vi "RT Main.vi"() -> ()   [LabVIEW 2021]
doc: "This example publishes data acquired from the myRIO device using shared variables. These shared variables can be accessed with an iPad running the sample dashboard."
uses:
  <vilib>/myRIO/Instrument Drivers/Utilities/Utilities.lvlib
  <vilib>/myRIO/Instrument Drivers/Onboard IO/AI/AI.lvlib
  <vilib>/myRIO/Instrument Drivers/Onboard IO/AO/AO.lvlib
  <vilib>/myRIO/Instrument Drivers/Onboard IO/DIO/DIO.lvlib
  <vilib>/ptbypt/NI_PtbyPt.lvlib
  <vilib>/Platform/TimedLoop/XDataNode/XDataNode.xnode
  <vilib>/Platform/TimedLoop/XDataNode/nitl_modes.ctl
  <vilib>/Platform/TimedLoop/XDataNode/XDNodeRunTimeDep.lvlib
  <vilib>/Platform/TimedLoop/XDataNode/wakeup.ctl
  <vilib>/Platform/TimedLoop/XDataNode/timing_clust.ctl
  <vilib>/myRIO/Instrument Drivers/Onboard IO/AI/vis/myRIO AI Open.xnode
  <vilib>/myRIO/Common/Instrument Driver Framework/Utilities/typedefs/Hardware Version Enum.ctl
  <vilib>/myRIO/Common/Instrument Driver Framework/Utilities/typedefs/Generic FPGA Reference.ctl
  <vilib>/myRIO/Common/Instrument Driver Framework/Utilities/typedefs/myRIO v1.0 Reference.ctl
  <vilib>/myRIO/Common/Instrument Driver Framework/Utilities/typedefs/myRIO Generic Hardware Reference.ctl
  <vilib>/myRIO/Common/Instrument Driver Framework/myRIO v1.0/AI/typedefs/AI Channels Enum.ctl
  <vilib>/myRIO/Common/Instrument Driver Framework/myRIO v1.0/AI/typedefs/AI Channels List.ctl
  <vilib>/myRIO/Common/Instrument Driver Framework/Utilities/typedefs/Analog Scaling Constants.ctl
  <vilib>/myRIO/Common/Instrument Driver Framework/Utilities/typedefs/Analog Scaling Constants List.ctl
  <vilib>/myRIO/Instrument Drivers/Onboard IO/AI/typedefs/AI Reference.ctl
  <vilib>/userdefined/High Color/nirio_resource_hc.ctl
  <vilib>/myRIO/Instrument Drivers/Onboard IO/AO/vis/myRIO AO Open.xnode
  <vilib>/myRIO/Common/Instrument Driver Framework/myRIO v1.0/AO/typedefs/AO Channels Enum.ctl
  <vilib>/myRIO/Common/Instrument Driver Framework/myRIO v1.0/AO/typedefs/AO Channels List.ctl
  <vilib>/myRIO/Instrument Drivers/Onboard IO/AO/typedefs/AO Reference.ctl
  <vilib>/myRIO/Instrument Drivers/Onboard IO/DIO/vis/myRIO DIO Open.xnode
  <vilib>/myRIO/Common/Instrument Driver Framework/myRIO v1.0/DIO/typedefs/DIO Channels Enum.ctl
  <vilib>/myRIO/Common/Instrument Driver Framework/myRIO v1.0/DIO/typedefs/DIO Channels List.ctl
  <vilib>/myRIO/Instrument Drivers/Onboard IO/DIO/typedefs/DIO Reference.ctl
  <vilib>/myRIO/Common/Instrument Driver Framework/myRIO v1.0/DIO/vis/myRIO v1.1 Open DIO.vi
  <vilib>/myRIO/Express VI/Onboard IO/AI/AI Express VI.xnode
  <vilib>/myRIO/Express VI/Onboard IO/AO/AO Express VI.xnode
  <vilib>/myRIO/Express VI/Onboard Devices/LED/LED Express VI.xnode
  <vilib>/myRIO/Common/Instrument Driver Framework/myRIO v1.0/AI/vis/myRIO v1.1 Open AI.vi
  <vilib>/myRIO/Common/Instrument Driver Framework/myRIO v1.0/AO/vis/myRIO v1.1 Open AO.vi
  <vilib>/myRIO/Common/Instrument Driver Framework/Utilities/vis/Is FPGA Ref Available.vi
  <vilib>/myRIO/Express VI/Onboard Devices/Accelerometer/Accelerometer Express VI.xnode
  <vilib>/myRIO/Instrument Drivers/Onboard Devices/Accelerometer/Accelerometer.lvlib
  <vilib>/myRIO/Common/Instrument Driver Framework/myRIO v1.0/Accelerometer/typedefs/Accelerometer Channels Enum.ctl
  <vilib>/myRIO/Common/Instrument Driver Framework/myRIO v1.0/Accelerometer/typedefs/Accelerometer Channels List.ctl
  <vilib>/myRIO/Instrument Drivers/Onboard Devices/Accelerometer/typedefs/Accelerometer Reference.ctl
  <vilib>/myRIO/Instrument Drivers/Onboard Devices/Accelerometer/vis/myRIO Accelerometer Open.xnode
  <vilib>/myRIO/Common/Instrument Driver Framework/myRIO v1.0/Accelerometer/vis/myRIO v1.1 Open Accelerometer.vi
panel:
  out "error out":errorcluster
  in  "stop":bool
  in  "Tab Control":T1(tab)
  out "LED3":bool
  out "LED2":bool
  out "LED1":bool
  out "LED0":bool
  out "Audio":waveform(dbl)[](graph)
  out "Accelerometer":waveform(dbl)[](graph)
  out "DIO.A":waveform(u8)(graph)
  out "AIO.A":waveform(dbl)[](graph)
  out "DIO.A Input/Output":enum16{"Input", "Output"}(ring)
  out "DIO Channel.A":u16(ring) items=["A/DIO0", "A/DIO1", "A/DIO2", "A/DIO3", "A/DIO4", "A/DIO5", "A/DIO6", "A/DIO7", "A/DIO8", "A/DIO9", "A/DIO10", "A/DIO11", "A/DIO12", "A/DIO13", "A/DIO14", "A/DIO15"]
  out "AO Channel.A":u16(ring) items=["A/AO0", "A/AO1"]
  out "AI Channel.A":u16(ring) items=["A/AI0", "A/AI1", "A/AI2", "A/AI3"]
  out "AIO.B":waveform(dbl)[](graph)
  out "DIO.B Input/Output":enum16{"Input", "Output"}(ring)
  out "DIO Channel.B":u16(ring) items=["B/DIO0", "B/DIO1", "B/DIO2", "B/DIO3", "B/DIO4", "B/DIO5", "B/DIO6", "B/DIO7", "B/DIO8", "B/DIO9", "B/DIO10", "B/DIO11", "B/DIO12", "B/DIO13", "B/DIO14", "B/DIO15"]
  out "AO Channel.B":u16(ring) items=["B/AO0", "B/AO1"]
  out "AI Channel.B":u16(ring) items=["B/AI0", "B/AI1", "B/AI2", "B/AI3"]
  out "DIO.B":waveform(u8)(graph)
  out "AIO.C":waveform(dbl)[](graph)
  out "DIO.C":waveform(u8)(graph)
  out "DIO.C Input/Output":enum16{"Input", "Output"}(ring)
  out "DIO Channel.C":u16(ring) items=["C/DIO0", "C/DIO1", "C/DIO2", "C/DIO3", "C/DIO4", "C/DIO5", "C/DIO6", "C/DIO7"]
  out "AO Channel.C":u16(ring) items=["C/AO0", "C/AO1"]
  out "AI Channel.C":u16(ring) items=["C/AI0", "C/AI1"]
  # "Overview: This example publishes data acquired from the myRIO device using shared variables.  These shared variables can be accessed with an iPad running the sample dashboard.\nRequirements: \n1. myRIO-1900\n2. Network Variable Engine on the myRIO\n3. Data Dashboard on iPad\nInstructions:\n1. Configure Data Dashboard for your iPad as described in the readme file for this project.  (Navigate to the Project Documentation folder in the project tree and open Data Dashboard for myRIO Readme.html.)\n2. Check the myRIO target IP Address in the project and make sure the target IP Address is correct.\n3. Run this VI."
  # "There are two ways to view the shared \nvariable data published by RT Main.vi that you\nrun on the myRIO:\n--View the data on iPad: You can find detailed \ninstructions in the readme file of the Data\nDashboard for myRIO example and the help file\nof Data Dashboard.\n--View the data on PC: Run RT Main.vi on the  \nmyRIO, and run Desktop Main.vi. View the \nshared variable data in Desktop Main.vi."
  # "LED Status :"
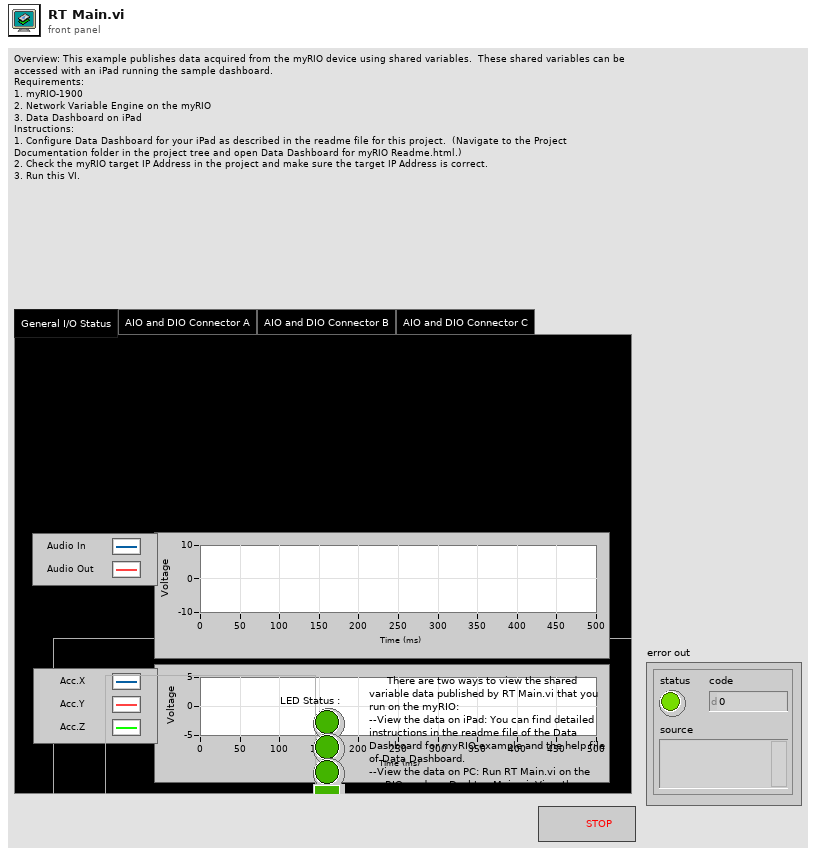
[diagram p1: front panel]
types:
  T1 = enum32{"General I/O Status", "AIO and DIO Connector A", "AIO and DIO Connector B", "AIO and DIO Connector C"}
  T2 = cluster{"read mode":enum16{"polling", "blocking"}, "write mode":enum16{"polling", "blocking"}}
  T3 = cluster{"AI.A":dbl, "AI.B":dbl, "AI.C":dbl, "AO.A":dbl, "AO.B":dbl, "AO.C":dbl, "DIO.A":u8, "DIO.B":u8, "DIO.C":u8, "Audio In":dbl, "Audio Out":dbl, "Accelerometer X":dbl, "Accelerometer Y":dbl, "Accelerometer Z":dbl, "LED0":bool, "LED1":bool, "LED2":bool, "LED3":bool}
  T4 = typedef "nirio_resource_hc.ctl" = tag
  T5 = typedef "Hardware Version Enum.ctl" = enum16{"Unknown", "myRIO-1900", "myRIO-1950", "roboRIO", "NI ELVIS RIO CM", "ELVIS III"}
  T6 = typedef "AO.lvlib/AO Reference.ctl" = cluster{"myRIO Reference":T7, "AO Channel List":T10, "AO Scaling Constant List":T12}
  T7 = typedef "myRIO Generic Hardware Reference.ctl" = cluster{"myRIO Model":T5, "myRIO Hardware Reference":T8}
  T8 = typedef "myRIO v1.0 Reference.ctl" = cluster{"Generic FPGA Reference":T9, "Allow multiple opens":bool}
  T9 = typedef "Generic FPGA Reference.ctl" = refnum<k20>
  T10 = typedef "AO Channels List.ctl" = T11[]
  T11 = typedef "AO Channels Enum.ctl" = enum16{"Not Connected", "AudioOut/Left", "AudioOut/Right", "C/AO0", "C/AO1", "A/AO0", "A/AO1", "B/AO0", "B/AO1"}
  T12 = typedef "Analog Scaling Constants List.ctl" = T13[]
  T13 = typedef "Analog Scaling Constants.ctl" = cluster{"LSB Weight (Volts)":dbl, "Offset (Volts)":dbl, "Signed?":bool}
  T14 = typedef "AI.lvlib/AI Reference.ctl" = cluster{"myRIO Reference":T7, "AI Channels List":T15, "AI Scaling Constants List":T12}
  T15 = typedef "AI Channels List.ctl" = T16[]
  T16 = typedef "AI Channels Enum.ctl" = enum16{"Not Connected", "AudioIn/Left", "AudioIn/Right", "C/AI0", "C/AI1", "A/AI0", "A/AI1", "A/AI2", "A/AI3", "A/AI4", "A/AI5", "A/AI6", "A/AI7", "B/AI0", "B/AI1", "B/AI2", "B/AI3", "B/AI4", "B/AI5", "B/AI6", "B/AI7", "AI/AI0", "AI/AI1", "AI/AI2", "AI/AI3", "A/AI0 (DIFF)", "A/AI1 (DIFF)", "A/AI2 (DIFF)", "A/AI3 (DIFF)", "B/AI0 (DIFF)", "B/AI1 (DIFF)", "B/AI2 (DIFF)", "B/AI3 (DIFF)"}
  T17 = typedef "Accelerometer.lvlib/Accelerometer Reference.ctl" = cluster{"myRIO Reference":T7, "Accelerometer Channels List":T18, "LSB Weight":dbl}
  T18 = typedef "Accelerometer Channels List.ctl" = T19[]
  T19 = typedef "Accelerometer Channels Enum.ctl" = enum16{"Not Connected", "X-Axis", "Y-Axis", "Z-Axis"}
  T20 = typedef "DIO.lvlib/DIO Reference.ctl" = cluster{"myRIO Reference":T7, "DIO Channels List":T21}
  T21 = typedef "DIO Channels List.ctl" = T22[]
  T22 = typedef "DIO Channels Enum.ctl" = enum16{"Not Connected", "C/DIO0", "C/DIO1", "C/DIO2", "C/DIO3", "C/DIO4", "C/DIO5", "C/DIO6", "C/DIO7", "A/DIO0", "A/DIO1", "A/DIO2", "A/DIO3", "A/DIO4", "A/DIO5", "A/DIO6", "A/DIO7", "A/DIO8", "A/DIO9", "A/DIO10", "A/DIO11", "A/DIO12", "A/DIO13", "A/DIO14", "A/DIO15", "A/DIO16", "A/DIO17", "A/DIO18", "A/DIO19", "B/DIO0", "B/DIO1", "B/DIO2", "B/DIO3", "B/DIO4", "B/DIO5", "B/DIO6", "B/DIO7", "B/DIO8", "B/DIO9", "B/DIO10", "B/DIO11", "B/DIO12", "B/DIO13", "B/DIO14", "B/DIO15", "B/DIO16", "B/DIO17", "B/DIO18", "B/DIO19", "LED0", "LED1", "LED2", "LED3", "Button0", "DIO/DIO0", "DIO/DIO1", "DIO/DIO2", "DIO/DIO3", "DIO/DIO4", "DIO/DIO5", "DIO/DIO6", "DIO/DIO7", "DIO/DIO8", "DIO/DIO9", "SPI/CS0", "SPI/CS1", "SPI/CS2", "SPI/CS3", "LED RADIO (Green)", "LED RADIO (Red)", "LED COMM (Green)", "LED COMM (Red)", "LED MODE (Green)", "LED MODE (Red)"}
  T23 = typedef "XDNodeRunTimeDep.lvlib/timing_clust.ctl" = cluster{"Expected End [f-1]":u64, "Actual End [f-1]":u64, "Finished Late? [f-1]":bool, "Expected End [i-1]":u64, "Actual End [i-1]":u64, "Finished Late? [i-1]":bool, "Expected Start [i]":u64, "Actual Start [i]":u64, "Expected Start [f]":u64, "Actual Start [f]":u64, "Source Name":string, "Structure Name":string, "Period":i64, "Deadline":i64, "Offset":i64, "Start":i64, "Priority":i32, "Timeout":i32, "Mode":T24, "Wakeup Reason":T25, "Error":errorcluster, "Source Type":string, "Secondary Source Type":string, "Global End Time":u64, "Global Start Time":u64, "Frame Duration":u64, "Iteration Duration":u64, "Assigned CPU":i32, "I/O Scan Engine Mode":u32}
  T24 = typedef "XDNodeRunTimeDep.lvlib/nitl_modes.ctl" = enum32{"No Change", "Process missed periods, maintain original phase", "Discard missed periods, maintain original phase", "Process missed periods, ignore original phase", "Discard missed periods, ignore original phase"}
  T25 = typedef "XDNodeRunTimeDep.lvlib/wakeup.ctl" = enum32{"Normal", "Aborted", "Asynchronous wakeup", "Timing source error", "Timed loop error", "Timeout"}
  T26 = cluster{"AI.A":dbl, "AI.B":dbl, "AI.C":dbl, "AO.A":dbl, "AO.B":dbl, "AO.C":dbl, "DIO.A":u8, "DIO.B":u8, "DIO.C":u8, "Audio In":dbl, "Audio Out":dbl, "Accelerometer X":dbl, "Accelerometer Y":dbl, "Accelerometer Z":dbl, "LED0":bool, "LED1":bool, "LED2":bool, "LED3":bool}[]
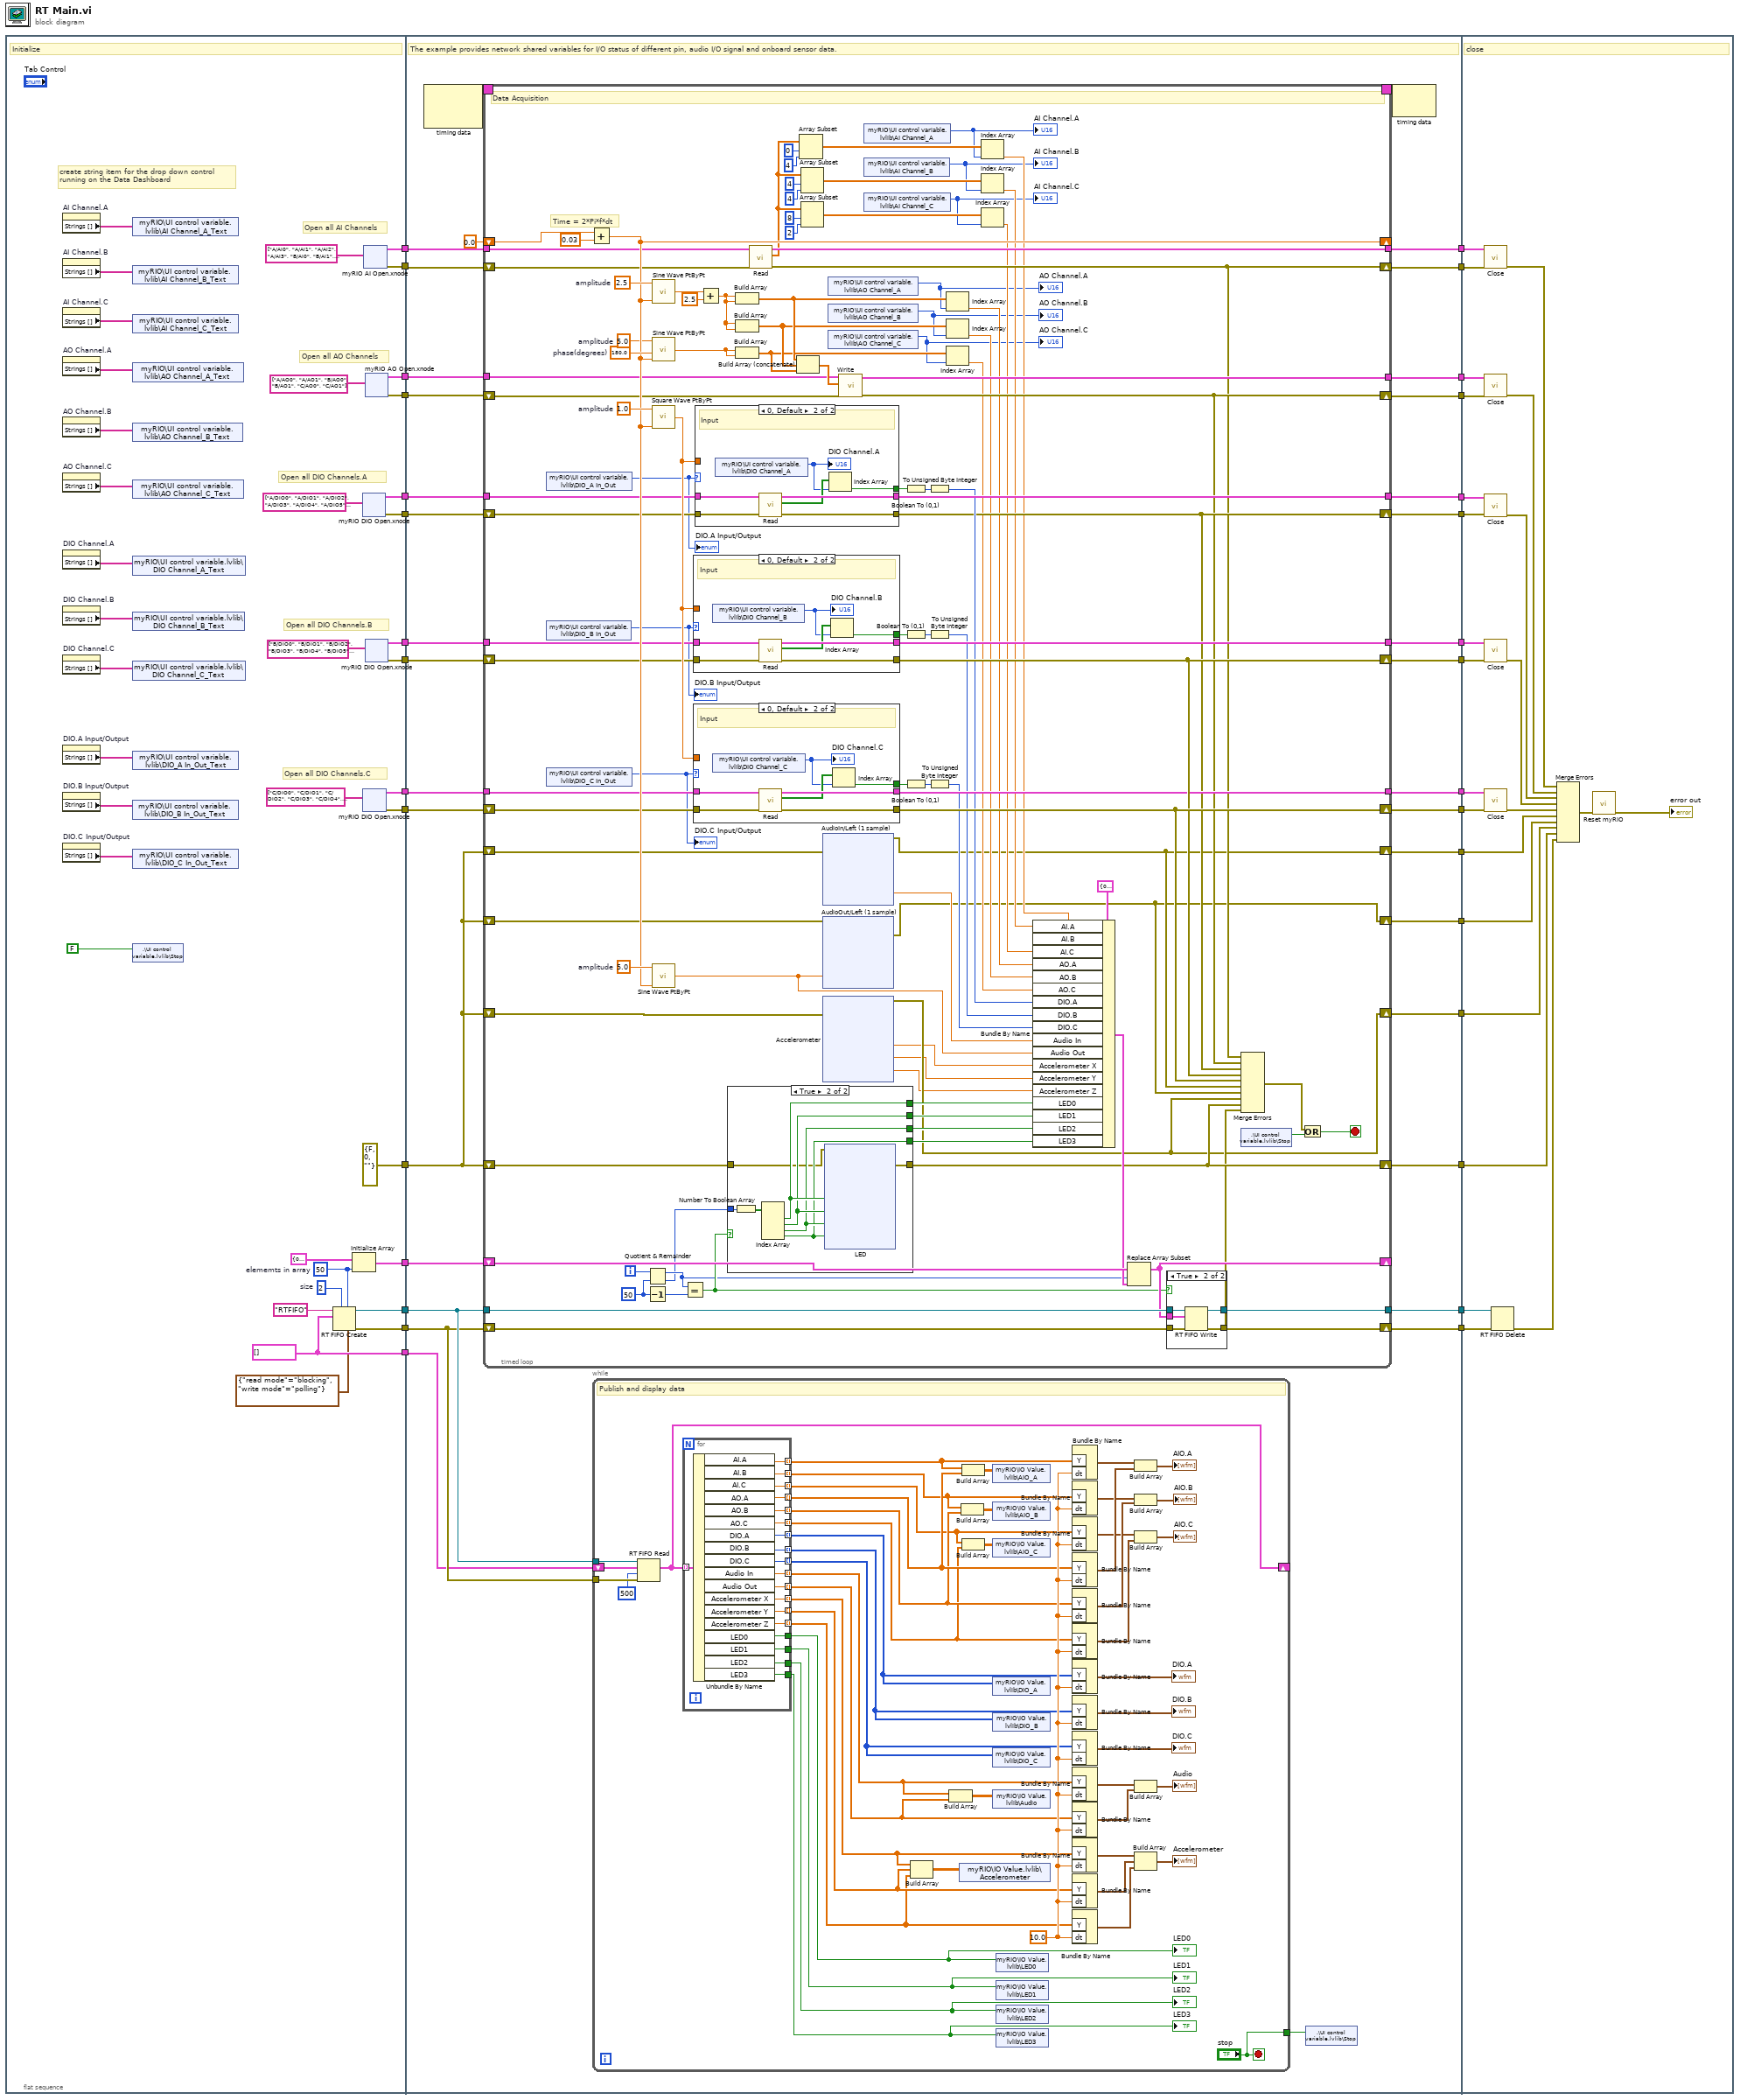
[diagram p0: block diagram]
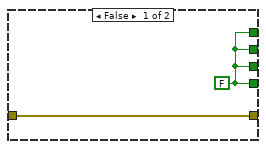
[diagram p2: hidden frame]
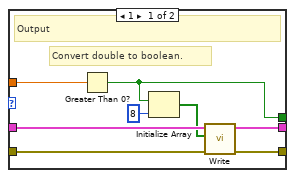
[diagram p4: hidden frame]
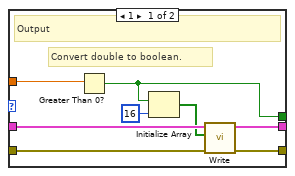
[diagram p5: hidden frame]
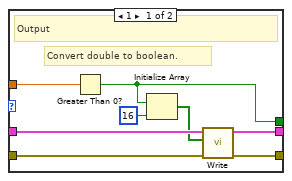
[diagram p6: hidden frame]
diagram:
  n1 = flat-sequence {
    tunnel: [errorcluster {"status"=FALSE, "code"=0, "source"=""} ("error IO")] -> w31
    tunnel: [w52] -> w14
    tunnel: [w51] -> w13
    tunnel: [w50] -> w12
    tunnel: [w49] -> w11
    tunnel: [w48] -> w10
    tunnel: [w47] -> w9
    tunnel: [w46] -> w8
    tunnel: [w45] -> w7
    tunnel: [w44] -> w6
    tunnel: [w43] -> w5
    tunnel: [w37] -> w4
    tunnel: [w36] -> w3
    tunnel: [w35] -> w2
    tunnel: [w34] -> w1
    tunnel: w31 -> [w161]
    tunnel: [w188] -> w30
    tunnel: [w155] -> w29
    tunnel: [w187] -> w28
    tunnel: [w184] -> w27
    tunnel: [w183] -> w26
    tunnel: [w182] -> w25
    tunnel: [w181] -> w24
    tunnel: [w180] -> w23
    tunnel: [w179] -> w22
    tunnel: [w178] -> w21
    tunnel: [w177] -> w20
    tunnel: [w176] -> w19
    tunnel: [w154] -> w18
    tunnel: [w175] -> w17
    tunnel: [w174] -> w16
    tunnel: [w172] -> w15
    tunnel: w14 -> [w166]
    tunnel: w13 -> [w171]
    tunnel: w12 -> [w170]
    tunnel: w11 -> [w169]
    tunnel: w10 -> [w168]
    tunnel: w9 -> [w167]
    tunnel: w8 -> [w165]
    tunnel: w7 -> [w164]
    tunnel: w6 -> [w163]
    tunnel: w5 -> [w162]
    tunnel: w4 -> [w157]
    tunnel: w3 -> [w160]
    tunnel: w2 -> [w159]
    tunnel: w1 -> [w158]
    tunnel: w30 -> [w596]
    tunnel: w29 -> [w602]
    tunnel: w28 -> [w601]
    tunnel: w27 -> [w595]
    tunnel: w26 -> [w592]
    tunnel: w25 -> [w593]
    tunnel: w24 -> [w590]
    tunnel: w23 -> [w589]
    tunnel: w22 -> [w586]
    tunnel: w21 -> [w587]
    tunnel: w20 -> [w584]
    tunnel: w19 -> [w583]
    tunnel: w18 -> [w600]
    tunnel: w17 -> [w599]
    tunnel: w16 -> [w598]
    tunnel: w15 -> [w581]
    frame #0 {
      w40 = u32 2  # size
      w39 = 50  # elememts in array
      w34 = T26 []
      # "Open all DIO Channels.C"
      # "Open all DIO Channels.B"
      # "Open all DIO Channels.A"
      # "Open all AO Channels"
      # "Open all AI Channels"
      # "create string item for the drop down control \nrunning on the Data Dashboard"
      # "Initialize"
      n2 = property on="AI Channel.A" class="Ring (strict)"() -> ("Strings []"=w69:string[])  [unwired: 2 in, 2 out]
      n3 = property on="AI Channel.B" class="Ring (strict)"() -> ("Strings []"=w68:string[])  [unwired: 2 in, 2 out]
      n4 = property on="AI Channel.C" class="Ring (strict)"() -> ("Strings []"=w67:string[])  [unwired: 2 in, 2 out]
      n5 = property on="AO Channel.A" class="Ring (strict)"() -> ("Strings []"=w66:string[])  [unwired: 2 in, 2 out]
      n6 = property on="AO Channel.B" class="Ring (strict)"() -> ("Strings []"=w65:string[])  [unwired: 2 in, 2 out]
      n7 = property on="AO Channel.C" class="Ring (strict)"() -> ("Strings []"=w64:string[])  [unwired: 2 in, 2 out]
      n8 = property on="DIO Channel.A" class="Ring (strict)"() -> ("Strings []"=w63:string[])  [unwired: 2 in, 2 out]
      n9 = property on="DIO Channel.B" class="Ring (strict)"() -> ("Strings []"=w62:string[])  [unwired: 2 in, 2 out]
      n10 = property on="DIO Channel.C" class="Ring (strict)"() -> ("Strings []"=w61:string[])  [unwired: 2 in, 2 out]
      n11 = property on="DIO.A Input/Output" class="Enum (strict)"() -> ("Strings []"=w60:string[])  [unwired: 2 in, 2 out]
      n12 = property on="DIO.B Input/Output" class="Enum (strict)"() -> ("Strings []"=w59:string[])  [unwired: 2 in, 2 out]
      n13 = property on="DIO.C Input/Output" class="Enum (strict)"() -> ("Strings []"=w58:string[])  [unwired: 2 in, 2 out]
      n14 = shared-variable "myRIO\\UI control variable.lvlib\\AI Channel_A_Text"(w69) -> ()  [unwired: 1 in, 1 out]
      n15 = shared-variable "myRIO\\UI control variable.lvlib\\AI Channel_B_Text"(w68) -> ()  [unwired: 1 in, 1 out]
      n16 = shared-variable "myRIO\\UI control variable.lvlib\\AI Channel_C_Text"(w67) -> ()  [unwired: 1 in, 1 out]
      n17 = shared-variable "myRIO\\UI control variable.lvlib\\AO Channel_A_Text"(w66) -> ()  [unwired: 1 in, 1 out]
      n18 = shared-variable "myRIO\\UI control variable.lvlib\\AO Channel_B_Text"(w65) -> ()  [unwired: 1 in, 1 out]
      n19 = shared-variable "myRIO\\UI control variable.lvlib\\AO Channel_C_Text"(w64) -> ()  [unwired: 1 in, 1 out]
      n20 = shared-variable "myRIO\\UI control variable.lvlib\\DIO Channel_A_Text"(w63) -> ()  [unwired: 1 in, 1 out]
      n21 = shared-variable "myRIO\\UI control variable.lvlib\\DIO Channel_B_Text"(w62) -> ()  [unwired: 1 in, 1 out]
      n22 = shared-variable "myRIO\\UI control variable.lvlib\\DIO Channel_C_Text"(w61) -> ()  [unwired: 1 in, 1 out]
      n23 = shared-variable "myRIO\\UI control variable.lvlib\\DIO_A In_Out_Text"(w60) -> ()  [unwired: 1 in, 1 out]
      n24 = shared-variable "myRIO\\UI control variable.lvlib\\DIO_B In_Out_Text"(w59) -> ()  [unwired: 1 in, 1 out]
      n25 = shared-variable "myRIO\\UI control variable.lvlib\\DIO_C In_Out_Text"(w58) -> ()  [unwired: 1 in, 1 out]
      n26 = shared-variable ".\\UI control variable.lvlib\\Stop"(FALSE ("End?")) -> ()  [unwired: 1 in, 1 out]
      n27 = RT FIFO Create(0:"RTFIFO" ("name (unnamed)"), 1:w34, 4:w40, 6:w39, 7:T2 {"read mode"=enum."blocking", "write mode"=enum."polling"} ("r/w modes (polling,polling)")) -> (8:w36:refnum<k33>, 11:w35:errorcluster)  [unwired: 3 in, 1 out]
      n28 = Initialize Array(T3 {"AI.A"=0.0, "AI.B"=0.0, "AI.C"=0.0, "AO.A"=0.0, "AO.B"=0.0, "AO.C"=0.0, "DIO.A"=0, "DIO.B"=0, "DIO.C"=0, "Audio In"=0.0, "Audio Out"=0.0, "Accelerometer X"=0.0, "Accelerometer Y"=0.0, "Accelerometer Z"=0.0, "LED0"=FALSE, "LED1"=FALSE, "LED2"=FALSE, "LED3"=FALSE}, w39) -> (w37:T26)
      n29 = xnode "myRIO DIO Open.xnode"("Channel Names"=tag[] ["A/DIO0", "A/DIO1", "A/DIO2", "A/DIO3", "A/DIO4", "A/DIO5", "A/DIO6", "A/DIO7", "A/DIO8", "A/DIO9", "A/DIO10", "A/DIO11", "A/DIO12", "A/DIO13", "A/DIO14", "A/DIO15"]) -> ("error out"=w45:errorcluster, "DIO Ref Out"=w49:T20)  [unwired: 2 in]
      n30 = xnode "myRIO DIO Open.xnode"("Channel Names"=tag[] ["C/DIO0", "C/DIO1", "C/DIO2", "C/DIO3", "C/DIO4", "C/DIO5", "C/DIO6", "C/DIO7"]) -> ("error out"=w43:errorcluster, "DIO Ref Out"=w47:T20)  [unwired: 2 in]
      n31 = xnode "myRIO AI Open.xnode"("Channel Names"=tag[] ["A/AI0", "A/AI1", "A/AI2", "A/AI3", "B/AI0", "B/AI1", "B/AI2", "B/AI3", "C/AI0", "C/AI1"]) -> ("error out"=w52:errorcluster, "AI Ref Out"=w51:T14)  [unwired: 2 in]
      n32 = xnode "myRIO AO Open.xnode"("Channel Names"=tag[] ["A/AO0", "A/AO1", "B/AO0", "B/AO1", "C/AO0", "C/AO1"]) -> ("error out"=w46:errorcluster, "AO Ref Out"=w50:T6)  [unwired: 2 in]
      n33 = xnode "myRIO DIO Open.xnode"("Channel Names"=tag[] ["B/DIO0", "B/DIO1", "B/DIO2", "B/DIO3", "B/DIO4", "B/DIO5", "B/DIO6", "B/DIO7", "B/DIO8", "B/DIO9", "B/DIO10", "B/DIO11", "B/DIO12", "B/DIO13", "B/DIO14", "B/DIO15"]) -> ("error out"=w44:errorcluster, "DIO Ref Out"=w48:T20)  [unwired: 2 in]
    }
    frame #1 {
      # "The example provides network shared variables for I/O status of different pin, audio I/O signal and onboard sensor data."
      n34 = node-c288() -> (w186:T23)  [unwired: 2 in]
      n35 = timed-loop {
        tunnel: [w277] -> w188
        shift-right: [w259] -> w184
        shift-left: w166 -> [w242]
        tunnel: [w276] -> w182
        shift-right: [w260] -> w183
        shift-left: w165 -> [w239]
        tunnel: [w275] -> w181
        tunnel: [w274] -> w179
        shift-right: [w292] -> w178
        shift-left: w163 -> [w235]
        shift-right: [w261] -> w180
        shift-left: w164 -> [w237]
        tunnel: [w273] -> w177
        shift-right: [w293] -> w176
        shift-left: w162 -> [w233]
        shift-right: [w193] -> w154
        shift-left: w161 -> [w194]
        shift-right: [w190] -> w175
        shift-left: w161 -> [w191]
        shift-right: [w198] -> w174
        shift-left: w161 -> [w199]
        shift-right: [w263] -> _
        shift-left: w157 -> [w269]
        tunnel: w160 -> [w264]
        shift-right: [w254] -> w187
        shift-left: w159 -> [w262]
        timing: w186 -> [_]
        timing-out: [_] -> w185
        shift-right: [w255] -> w172
        shift-left: w161 -> [w256]
        shift-right: [w244] -> _
        shift-left: 0.0 -> [w246]
        tunnel: w171 -> [w241]
        tunnel: w170 -> [w240]
        tunnel: w169 -> [w238]
        tunnel: w168 -> [w236]
        tunnel: w167 -> [w234]
        tunnel: [w209] -> w155
        i -> [w268]
        stop <- w289 stop-if-true
        w243 = 5.0  # amplitude
        w257 = 5.0  # amplitude
        w267 = 50 ("y")
        w287 = 2.5  # amplitude
        w288 = 180.0  # phase(degrees)
        w290 = 1.0  # amplitude
        # "Time = 2*Pi*f*dt"
        # "Data Acquisition"
        n36 = shared-variable "myRIO\\UI control variable.lvlib\\DIO_A In_Out"() -> (w202:u16)  [unwired: 1 in, 1 out]
        "DIO.A Input/Output" <- w202
        n37 = shared-variable "myRIO\\UI control variable.lvlib\\DIO_B In_Out"() -> (w200:u16)  [unwired: 1 in, 1 out]
        "DIO.B Input/Output" <- w200
        n38 = shared-variable "myRIO\\UI control variable.lvlib\\DIO_C In_Out"() -> (w201:u16)  [unwired: 1 in, 1 out]
        "DIO.C Input/Output" <- w201
        n39 = Add(x=w246, y=0.03) -> (x+y=w244:dbl)
        n40 = Decrement(x=w267) -> (x-1=w266:i32)
        n41 = Quotient & Remainder(x=w268, y=w267) -> (x-y*floor(x/y)=w252:i32, floor(x/y)=w251:i32)
        n42 = call <vilib>:"Sine Wave PtByPt.vi"("time"=w244, "amplitude"=w287) -> ("sine wave"=w285:dbl)  [unwired: 2 in]
        n43 = call <vilib>:"Sine Wave PtByPt.vi"("time"=w244, "phase"=w288, "amplitude"=w243) -> ("sine wave"=w216:dbl)  [unwired: 1 in]
        n44 = call <vilib>:"Square Wave PtByPt.vi"("amplitude"=w290, "time"=w244) -> ("square wave"=w291:dbl)  [unwired: 3 in]
        n45 = call <vilib>:"Sine Wave PtByPt.vi"("time"=w244, "amplitude"=w257) -> ("sine wave"=w189:dbl)  [unwired: 2 in]
        n46 = Equal?(x=w252, y=w266) -> (x = y?=w253:bool)
        n47 = case shown="0, Default" w200 {
          tunnel: w236 -> [w482 w491]
          tunnel: w235 -> [w481 w490]
          tunnel: [w484 w489] -> w274
          tunnel: [w483 w488] -> w292
          tunnel: [w478 w486] -> w279
          tunnel: w291 -> [w479 _]
          frame 1 {
            # "Convert double to boolean."
            # "Output"
            n48 = Greater Than 0?(x=w479) -> (x > 0?=w478:bool)
            n49 = Initialize Array(w478, 16 ("dimension size")) -> (w477:bool[])
            n50 = call <vilib>:"Write.vi"("error in (no error)"=w481, "Values"=w477, "DIO Ref In"=w482) -> ("error out"=w483:errorcluster, "DIO Ref Out"=w484:T20)  [unwired: 6 in]
          }
          frame 0, Default {
            # "Input"
            n51 = shared-variable "myRIO\\UI control variable.lvlib\\DIO Channel_B"() -> (w485:u16)  [unwired: 1 in, 1 out]
            "DIO Channel.B" <- w485
            n52 = call <vilib>:"Read.vi"("error in (no error)"=w490, "DIO Ref In"=w491) -> ("error out"=w488:errorcluster, "Values"=w487:bool[], "DIO Ref Out"=w489:T20)  [unwired: 7 in]
            n53 = Index Array(array=w487, index=w485) -> (element=w486:bool)
          }
        }
        n54 = case shown="0, Default" w201 {
          tunnel: w234 -> [w467 w476]
          tunnel: w233 -> [w466 w475]
          tunnel: [w469 w474] -> w273
          tunnel: [w468 w473] -> w293
          tunnel: [w463 w471] -> w278
          tunnel: w291 -> [w465 _]
          frame 1 {
            # "Convert double to boolean."
            # "Output"
            n55 = Greater Than 0?(x=w465) -> (x > 0?=w463:bool)
            n56 = Initialize Array(w463, 8 ("dimension size")) -> (w462:bool[])
            n57 = call <vilib>:"Write.vi"("error in (no error)"=w466, "Values"=w462, "DIO Ref In"=w467) -> ("error out"=w468:errorcluster, "DIO Ref Out"=w469:T20)  [unwired: 6 in]
          }
          frame 0, Default {
            # "Input"
            n58 = shared-variable "myRIO\\UI control variable.lvlib\\DIO Channel_C"() -> (w470:u16)  [unwired: 1 in, 1 out]
            "DIO Channel.C" <- w470
            n59 = call <vilib>:"Read.vi"("error in (no error)"=w475, "DIO Ref In"=w476) -> ("error out"=w473:errorcluster, "Values"=w472:bool[], "DIO Ref Out"=w474:T20)  [unwired: 7 in]
            n60 = Index Array(array=w472, index=w470) -> (element=w471:bool)
          }
        }
        n61 = case shown="0, Default" w202 {
          tunnel: w238 -> [w497 w506]
          tunnel: w237 -> [w496 w505]
          tunnel: [w499 w504] -> w275
          tunnel: [w498 w503] -> w261
          tunnel: [w494 w501] -> w283
          tunnel: w291 -> [w492 _]
          frame 1 {
            # "Convert double to boolean."
            # "Output"
            n62 = Greater Than 0?(x=w492) -> (x > 0?=w494:bool)
            n63 = Initialize Array(w494, 16 ("dimension size")) -> (w493:bool[])
            n64 = call <vilib>:"Write.vi"("error in (no error)"=w496, "Values"=w493, "DIO Ref In"=w497) -> ("error out"=w498:errorcluster, "DIO Ref Out"=w499:T20)  [unwired: 6 in]
          }
          frame 0, Default {
            # "Input"
            n65 = shared-variable "myRIO\\UI control variable.lvlib\\DIO Channel_A"() -> (w500:u16)  [unwired: 1 in, 1 out]
            "DIO Channel.A" <- w500
            n66 = call <vilib>:"Read.vi"("error in (no error)"=w505, "DIO Ref In"=w506) -> ("error out"=w503:errorcluster, "Values"=w502:bool[], "DIO Ref Out"=w504:T20)  [unwired: 7 in]
            n67 = Index Array(array=w502, index=w500) -> (element=w501:bool)
          }
        }
        n68 = Add(x=w285, y=2.5) -> (x+y=w219:dbl)
        n69 = case shown="True" w253 {
          tunnel: w256 -> [w408 w409]
          tunnel: [w408 w410] -> w255
          tunnel: w251 -> [_ w416]
          tunnel: [w407 w414] -> w250
          tunnel: [w407 w413] -> w249
          tunnel: [w407 w412] -> w248
          tunnel: [w407 w411] -> w247
          frame False {
            w407 = FALSE
          }
          frame True {
            n70 = Number To Boolean Array(number=w416) -> (Boolean array=w415:bool[])
            n71 = Index Array(array=w415) -> (element #1=w414:bool, element #2=w413:bool, element #3=w412:bool, element #4=w411:bool)  [unwired: 4 in]
            n72 = xnode "LED"("LED0"=w414, "LED1"=w413, "LED2"=w412, "LED3"=w411, "error in (no error)"=w409) -> ("error out"=w410:errorcluster)
          }
        }
        n73 = Build Array(w219, w219) -> (w214:dbl[])
        n74 = Build Array(w219, w219) -> (w213:dbl[])
        n75 = Build Array(w216, w216) -> (w212:dbl[])
        n76 = call <vilib>:"Read.vi"("error in (no error)"=w242, "AI Ref In"=w241) -> ("error out"=w259:errorcluster, "Values"=w226:dbl[], "AI Ref Out"=w277:T14)  [unwired: 7 in]
        n77 = Build Array (concatenate)(w214, w213, w212) -> (w280:dbl[])
        n78 = Array Subset(array=w226, index=0, length=4) -> (w225:dbl[])
        n79 = Array Subset(array=w226, index=4, length=4) -> (w223:dbl[])
        n80 = Array Subset(array=w226, index=8, length=2) -> (w221:dbl[])
        n81 = xnode "AudioIn/Left (1 sample)"("error in (no error)"=w194) -> ("AudioIn/Left"=w192:dbl, "error out"=w193:errorcluster)
        n82 = xnode "AudioOut/Left (1 sample)"("AudioOut/Left"=w189, "error in (no error)"=w191) -> ("error out"=w190:errorcluster)
        n83 = xnode "Accelerometer"("error in (no error)"=w199) -> ("X-Axis"=w197:dbl, "Y-Axis"=w196:dbl, "Z-Axis"=w195:dbl, "error out"=w198:errorcluster)
        n84 = shared-variable "myRIO\\UI control variable.lvlib\\AO Channel_A"() -> (w205:u16)  [unwired: 1 in, 1 out]
        "AO Channel.A" <- w205
        n85 = shared-variable "myRIO\\UI control variable.lvlib\\AO Channel_B"() -> (w204:u16)  [unwired: 1 in, 1 out]
        "AO Channel.B" <- w204
        n86 = shared-variable "myRIO\\UI control variable.lvlib\\AO Channel_C"() -> (w203:u16)  [unwired: 1 in, 1 out]
        "AO Channel.C" <- w203
        n87 = call <vilib>:"Write.vi"("error in (no error)"=w239, "Values"=w280, "AO Ref In"=w240) -> ("error out"=w260:errorcluster, "AO Ref Out"=w276:T6)  [unwired: 6 in]
        n88 = shared-variable "myRIO\\UI control variable.lvlib\\AI Channel_A"() -> (w208:u16)  [unwired: 1 in, 1 out]
        "AI Channel.A" <- w208
        n89 = shared-variable "myRIO\\UI control variable.lvlib\\AI Channel_B"() -> (w207:u16)  [unwired: 1 in, 1 out]
        "AI Channel.B" <- w207
        n90 = shared-variable "myRIO\\UI control variable.lvlib\\AI Channel_C"() -> (w206:u16)  [unwired: 1 in, 1 out]
        "AI Channel.C" <- w206
        n91 = Boolean To (0,1)(Boolean=w283) -> (0, 1=w284:i16)
        n92 = Boolean To (0,1)(Boolean=w279) -> (0, 1=w282:i16)
        n93 = Boolean To (0,1)(Boolean=w278) -> (0, 1=w281:i16)
        n94 = To Unsigned Byte Integer(number=w284) -> (unsigned 8bit integer=w272:u8)
        n95 = To Unsigned Byte Integer(number=w282) -> (unsigned 8bit integer=w271:u8)
        n96 = To Unsigned Byte Integer(number=w281) -> (unsigned 8bit integer=w270:u8)
        n97 = Index Array(array=w214, index=w205) -> (element=w218:dbl)
        n98 = Index Array(array=w213, index=w204) -> (element=w217:dbl)
        n99 = Index Array(array=w212, index=w203) -> (element=w215:dbl)
        n100 = Index Array(array=w225, index=w208) -> (element=w224:dbl)
        n101 = Index Array(array=w223, index=w207) -> (element=w222:dbl)
        n102 = Index Array(array=w221, index=w206) -> (element=w220:dbl)
        n103 = Bundle By Name(cluster=T3 {"AI.A"=0.0, "AI.B"=0.0, "AI.C"=0.0, "AO.A"=0.0, "AO.B"=0.0, "AO.C"=0.0, "DIO.A"=0, "DIO.B"=0, "DIO.C"=0, "Audio In"=0.0, "Audio Out"=0.0, "Accelerometer X"=0.0, "Accelerometer Y"=0.0, "Accelerometer Z"=0.0, "LED0"=FALSE, "LED1"=FALSE, "LED2"=FALSE, "LED3"=FALSE}, "AI.A"=w224, "AI.B"=w222, "AI.C"=w220, "AO.A"=w218, "AO.B"=w217, "AO.C"=w215, "DIO.A"=w272, "DIO.B"=w271, "DIO.C"=w270, "Audio In"=w192, "Audio Out"=w189, "Accelerometer X"=w197, "Accelerometer Y"=w196, "Accelerometer Z"=w195, "LED0"=w250, "LED1"=w249, "LED2"=w248, "LED3"=w247) -> (w265:T3)
        n104 = Replace Array Subset(array=w269, new element=w265, index=w252) -> (w263:T26)
        n105 = case shown="True" w253 {
          tunnel: w264 -> [w455 w461]
          tunnel: w263 -> [_ w460]
          tunnel: w262 -> [w456 w459]
          tunnel: [w456 w458] -> w254
          tunnel: [w455 w457] -> w209
          frame False {
          }
          frame True {
            n106 = RT FIFO Write(0:w461, 1:w460, 3:w459) -> (8:w457:refnum<k33>, 11:w458:errorcluster)  [unwired: 2 in, 2 out]
          }
        }
        n107 = shared-variable ".\\UI control variable.lvlib\\Stop"() -> (w210:bool)  [unwired: 1 in, 1 out]
        n108 = Merge Errors(w259, w260, w261, w292, w293, w193, w190, w198, w255, w254) -> (w258:errorcluster)
        n109 = Or(x=w258, y=w210) -> (x .or. y?=w289:bool)
      }
      n110 = while {
        tunnel: w160 -> [w557]
        tunnel: w159 -> [w556]
        shift-right: [w546] -> _
        shift-left: w158 -> [w548]
        tunnel: ["stop"] -> w156
        stop <- "stop" stop-if-true
        w559 = 10.0 ("dt")
        # "Publish and display data"
        n111 = RT FIFO Read(0:w557, 1:w548, 2:500 ("timeout in ms (0)"), 3:w556) -> (9:w546:T26)  [unwired: 4 out]
        n112 = for {
          tunnel: w546 -> [w578] mode=indexing
          tunnel: [w577] -> w533 mode=indexing
          tunnel: [w576] -> w530 mode=indexing
          tunnel: [w575] -> w527 mode=indexing
          tunnel: [w574] -> w531 mode=indexing
          tunnel: [w573] -> w529 mode=indexing
          tunnel: [w572] -> w526 mode=indexing
          tunnel: [w571] -> w555 mode=indexing
          tunnel: [w570] -> w554 mode=indexing
          tunnel: [w569] -> w553 mode=indexing
          tunnel: [w568] -> w524 mode=indexing
          tunnel: [w567] -> w523 mode=indexing
          tunnel: [w566] -> w520 mode=indexing
          tunnel: [w565] -> w519 mode=indexing
          tunnel: [w564] -> w518 mode=indexing
          tunnel: [w563] -> w552
          tunnel: [w562] -> w551
          tunnel: [w561] -> w550
          tunnel: [w560] -> w549
          n113 = Unbundle By Name(w578) -> ("AI.A"=w577:dbl, "AI.B"=w576:dbl, "AI.C"=w575:dbl, "AO.A"=w574:dbl, "AO.B"=w573:dbl, "AO.C"=w572:dbl, "DIO.A"=w571:u8, "DIO.B"=w570:u8, "DIO.C"=w569:u8, "Audio In"=w568:dbl, "Audio Out"=w567:dbl, "Accelerometer X"=w566:dbl, "Accelerometer Y"=w565:dbl, "Accelerometer Z"=w564:dbl, "LED0"=w563:bool, "LED1"=w562:bool, "LED2"=w561:bool, "LED3"=w560:bool)
        }
        "LED0" <- w552
        "LED1" <- w551
        "LED2" <- w550
        "LED3" <- w549
        n114 = Build Array(w520, w519, w518) -> (w521:dbl[][])
        n115 = Build Array(w524, w523) -> (w522:dbl[][])
        n116 = shared-variable "myRIO\\IO Value.lvlib\\Accelerometer"(w521) -> ()  [unwired: 1 in, 1 out]
        n117 = Build Array(w530, w529) -> (w528:dbl[][])
        n118 = Build Array(w533, w531) -> (w532:dbl[][])
        n119 = Build Array(w527, w526) -> (w525:dbl[][])
        n120 = shared-variable "myRIO\\IO Value.lvlib\\AIO_A"(w532) -> ()  [unwired: 1 in, 1 out]
        n121 = shared-variable "myRIO\\IO Value.lvlib\\AIO_C"(w525) -> ()  [unwired: 1 in, 1 out]
        n122 = shared-variable "myRIO\\IO Value.lvlib\\DIO_A"(w555) -> ()  [unwired: 1 in, 1 out]
        n123 = shared-variable "myRIO\\IO Value.lvlib\\DIO_C"(w553) -> ()  [unwired: 1 in, 1 out]
        n124 = shared-variable "myRIO\\IO Value.lvlib\\AIO_B"(w528) -> ()  [unwired: 1 in, 1 out]
        n125 = shared-variable "myRIO\\IO Value.lvlib\\DIO_B"(w554) -> ()  [unwired: 1 in, 1 out]
        n126 = shared-variable "myRIO\\IO Value.lvlib\\Audio"(w522) -> ()  [unwired: 1 in, 1 out]
        n127 = shared-variable "myRIO\\IO Value.lvlib\\LED0"(w552) -> ()  [unwired: 1 in, 1 out]
        n128 = shared-variable "myRIO\\IO Value.lvlib\\LED1"(w551) -> ()  [unwired: 1 in, 1 out]
        n129 = shared-variable "myRIO\\IO Value.lvlib\\LED2"(w550) -> ()  [unwired: 1 in, 1 out]
        n130 = shared-variable "myRIO\\IO Value.lvlib\\LED3"(w549) -> ()  [unwired: 1 in, 1 out]
        n131 = Bundle By Name("Y"=w533, "dt"=w559) -> (w545:waveform(dbl))  [unwired: 1 in]
        n132 = Bundle By Name("Y"=w530, "dt"=w559) -> (w542:waveform(dbl))  [unwired: 1 in]
        n133 = Bundle By Name("Y"=w527, "dt"=w559) -> (w540:waveform(dbl))  [unwired: 1 in]
        n134 = Bundle By Name("Y"=w531, "dt"=w559) -> (w544:waveform(dbl))  [unwired: 1 in]
        n135 = Bundle By Name("Y"=w529, "dt"=w559) -> (w541:waveform(dbl))  [unwired: 1 in]
        n136 = Bundle By Name("Y"=w526, "dt"=w559) -> (w539:waveform(dbl))  [unwired: 1 in]
        n137 = Bundle By Name("Y"=w555, "dt"=w559) -> (→"DIO.A":waveform(u8))  [unwired: 1 in]
        n138 = Bundle By Name("Y"=w554, "dt"=w559) -> (→"DIO.B":waveform(u8))  [unwired: 1 in]
        n139 = Bundle By Name("Y"=w553, "dt"=w559) -> (→"DIO.C":waveform(u8))  [unwired: 1 in]
        n140 = Bundle By Name("Y"=w524, "dt"=w559) -> (w538:waveform(dbl))  [unwired: 1 in]
        n141 = Bundle By Name("Y"=w523, "dt"=w559) -> (w537:waveform(dbl))  [unwired: 1 in]
        n142 = Bundle By Name("Y"=w520, "dt"=w559) -> (w536:waveform(dbl))  [unwired: 1 in]
        n143 = Bundle By Name("Y"=w519, "dt"=w559) -> (w535:waveform(dbl))  [unwired: 1 in]
        n144 = Bundle By Name("Y"=w518, "dt"=w559) -> (w534:waveform(dbl))  [unwired: 1 in]
        n145 = Build Array(w545, w544) -> (→"AIO.A":waveform(dbl)[])
        n146 = Build Array(w542, w541) -> (→"AIO.B":waveform(dbl)[])
        n147 = Build Array(w540, w539) -> (→"AIO.C":waveform(dbl)[])
        n148 = Build Array(w538, w537) -> (→"Audio":waveform(dbl)[])
        n149 = Build Array(w536, w535, w534) -> (→"Accelerometer":waveform(dbl)[])
      }
      n150 = shared-variable ".\\UI control variable.lvlib\\Stop"(w156) -> ()  [unwired: 1 in, 1 out]
      n151 = node-c288(w185) -> ()  [unwired: 1 out]
    }
    frame #2 {
      # "close"
      n152 = call <vilib>:"Close.vi"("error in (no error)"=w595, "AI Ref In"=w596) -> ("error out"=w594:errorcluster)  [unwired: 9 in]
      n153 = call <vilib>:"Close.vi"("error in (no error)"=w592, "AO Ref In"=w593) -> ("error out"=w591:errorcluster)  [unwired: 9 in]
      n154 = call <vilib>:"Close.vi"("error in (no error)"=w589, "DIO Ref In"=w590) -> ("error out"=w588:errorcluster)  [unwired: 9 in]
      n155 = call <vilib>:"Close.vi"("error in (no error)"=w587, "DIO Ref In"=w586) -> ("error out"=w585:errorcluster)  [unwired: 9 in]
      n156 = call <vilib>:"Close.vi"("error in (no error)"=w583, "DIO Ref In"=w584) -> ("error out"=w582:errorcluster)  [unwired: 9 in]
      n157 = RT FIFO Delete(0:w602, 3:w601) -> (11:w580:errorcluster)  [unwired: 1 in]
      n158 = Merge Errors(w594, w591, w588, w585, w582, w600, w599, w598, w581, w580) -> (w597:errorcluster)
      n159 = call <vilib>:"Reset myRIO.vi"("error in (no error)"=w597) -> ("error out"=→"error out":errorcluster)  [unwired: 10 in]
    }
  }
